vi "Request - Parse Header.vi"() -> (3 "Unit Test Framework Results":T1)   [LabVIEW 2023, in "Request.lvclass"]
doc: "Use this template to create a user-defined test VI. Define your test requirements and wire the results to the <b>Result (Test)</b> control. Do not modify the <b>Unit Test Framework Results</b> indicator."
uses:
  Request.lvclass
  <vilib>/utf/common/utf_test_comparison_operators.ctl
  <vilib>/utf/NI_UnitTestFramework.lvlib
  <vilib>/utf/common/utf_test_result.ctl
  <vilib>/utf/common/utf_test_result_failure.ctl
  <vilib>/utf/common/utf_test_result_troll.ctl
  <vilib>/utf/common/utf_vi_tag.ctl
  Request.ctl
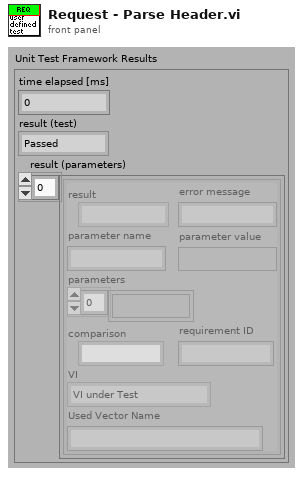
[diagram p1: front panel]
types:
  T1 = typedef "NI_UnitTestFramework.lvlib/utf_test_result_troll.ctl" = cluster{"time elapsed [ms]":u32, "result (test)":T2, "result (parameters)":T3[]}
  T2 = typedef "NI_UnitTestFramework.lvlib/utf_test_result.ctl" = enum16{"Passed", "Failed", "Error", "Skipped", "Not Processed"}
  T3 = typedef "NI_UnitTestFramework.lvlib/utf_test_result_failure.ctl" = cluster{"result":T2, "error message":string, "parameter name":string, "parameter value":variant, "parameters":variant[], "comparison":T4, "requirement ID":string, "VI":T5, "Used Vector Name":string}
  T4 = typedef "NI_UnitTestFramework.lvlib/utf_test_comparison_operators.ctl" = enum16{"=", "!=", ">", ">=", "<", "<=", "range", "symmetric tolerance", "asymmetric tolerance", "string contains", "string not contain", "array size", "string length", "array range", "by element", "array range (limit array)", "user-defined", "array contains", "array not contain", "vector length", "= (elm)", "!= (elm)", "= (case insensitive)", "!= (case insensitive)"}
  T5 = typedef "NI_UnitTestFramework.lvlib/utf_vi_tag.ctl" = enum16{"Setup VI", "VI under Test", "Teardown VI"}
  T6 = typedef "Request.ctl" = cluster{"Method":string, "URI":string, "Protocol":string, "Raw Path":string, "Query":string, "Fragment":string, "Raw Body":string, "Headers":variant, "Parameters":variant, "Body":variant, "Raw Header":string, "Path":string[]}
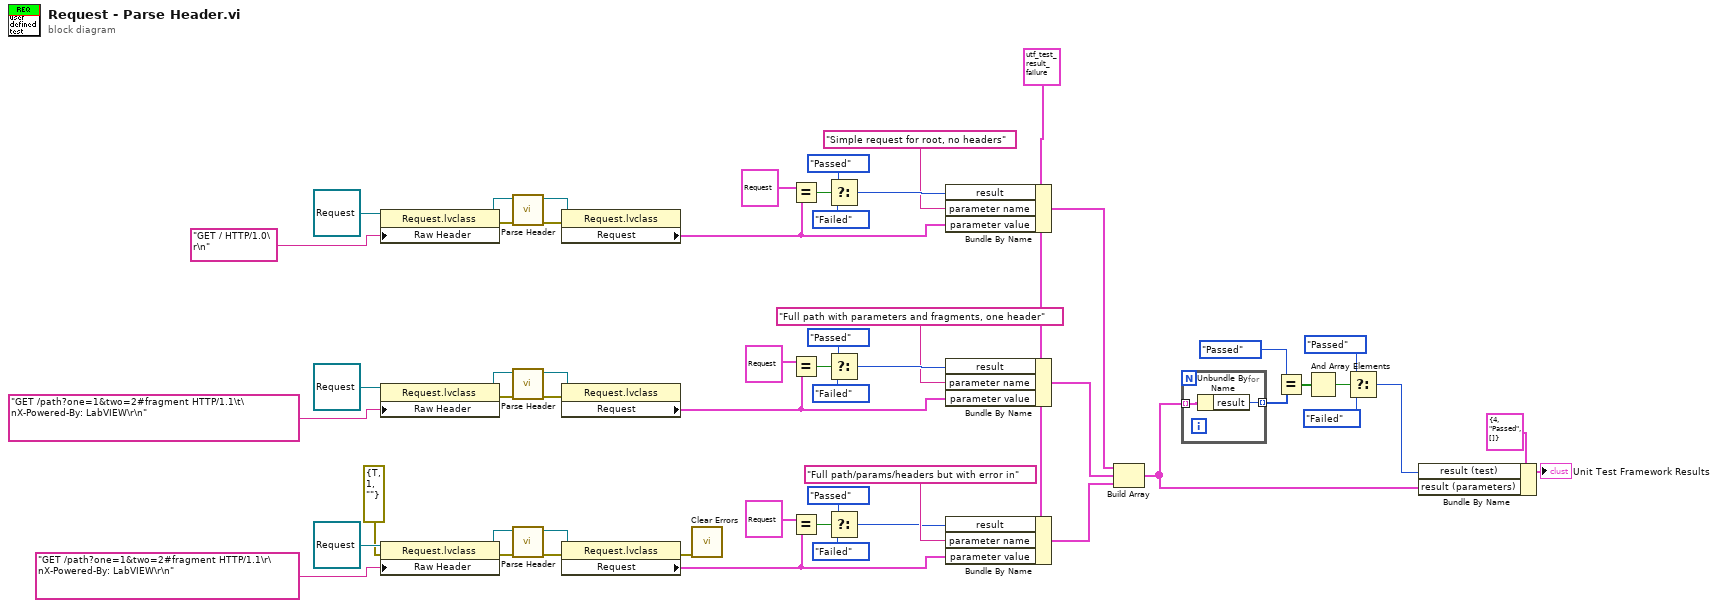
[diagram p0: block diagram]
diagram:
  w9 = T3 {"result"=enum."Not Processed", "error message"="", "parameter name"="", "parameter value"=variant, "parameters"=[], "comparison"=enum."=", "requirement ID"="", "VI"=enum."VI under Test", "Used Vector Name"=""} ("Unit Test Framework - result (parameters)")
  n1 = property class="Request.lvclass"(reference=refnum<class "Request.lvclass"> refnum ("Request.lvclass"), "Raw Header"="GET / HTTP/1.0\r\n") -> (reference out=w52:refnum<class "Request.lvclass">, error out=w51:errorcluster)  [unwired: 1 in]
  n2 = property class="Request.lvclass"(reference=refnum<class "Request.lvclass"> refnum ("Request.lvclass"), "Raw Header"="GET /path?one=1&two=2#fragment HTTP/1.1\t\nX-Powered-By: LabVIEW\r\n") -> (reference out=w30:refnum<class "Request.lvclass">, error out=w31:errorcluster)  [unwired: 1 in]
  n3 = property class="Request.lvclass"(reference=refnum<class "Request.lvclass"> refnum ("Request.lvclass"), error in=errorcluster {"status"=TRUE, "code"=1, "source"=""} ("error in (no error)"), "Raw Header"="GET /path?one=1&two=2#fragment HTTP/1.1\r\nX-Powered-By: LabVIEW\r\n") -> (reference out=w15:refnum<class "Request.lvclass">, error out=w14:errorcluster)
  n4 = call "Parse Header.vi"("error in (no error)"=w51, "Request in"=w52) -> ("error out"=w50:errorcluster, "Request out"=w49:refnum<class "Request.lvclass">)  [unwired: 8 in]
  n5 = call "Parse Header.vi"("error in (no error)"=w31, "Request in"=w30) -> ("error out"=w32:errorcluster, "Request out"=w33:refnum<class "Request.lvclass">)  [unwired: 8 in]
  n6 = call "Parse Header.vi"("error in (no error)"=w14, "Request in"=w15) -> ("error out"=w13:errorcluster, "Request out"=w12:refnum<class "Request.lvclass">)  [unwired: 8 in]
  n7 = property class="Request.lvclass"(reference=w49, error in=w50) -> ("Request"=w4:T6)  [unwired: 2 out]
  n8 = property class="Request.lvclass"(reference=w33, error in=w32) -> ("Request"=w6:T6)  [unwired: 2 out]
  n9 = property class="Request.lvclass"(reference=w12, error in=w13) -> (error out=w7:errorcluster, "Request"=w5:T6)  [unwired: 1 out]
  n10 = call <vilib>:"Clear Errors.vi"("error in (no error)"=w7) -> ()  [unwired: 5 in, 2 out]
  n11 = Equal?(x=T6 {"Method"="GET", "URI"="/", "Protocol"="HTTP/1.0", "Raw Path"="/", "Query"="", "Fragment"="", "Raw Body"="", "Headers"=variant, "Parameters"=variant, "Body"=variant, "Raw Header"="GET / HTTP/1.0\r\n", "Path"=[""]} ("Request"), y=w4) -> (x = y?=w35:bool)
  n12 = Equal?(x=T6 {"Method"="GET", "URI"="/path?one=1&two=2#fragment", "Protocol"="HTTP/1.1\t\nX-Powered-By:", "Raw Path"="/path?one=1&two=2", "Query"="one=1&two=2", "Fragment"="fragment", "Raw Body"="", "Headers"=variant, "Parameters"=variant("one"=variant(string "1"), "two"=variant(string "2")), "Body"=variant, "Raw Header"="GET /path?one=1&two=2#fragment HTTP/1.1\t\nX-Powered-By: LabVIEW\r\n", "Path"=["path"]} ("Request 2"), y=w6) -> (x = y?=w28:bool)
  n13 = Equal?(x=T6 {"Method"="", "URI"="", "Protocol"="", "Raw Path"="", "Query"="", "Fragment"="", "Raw Body"="", "Headers"=variant, "Parameters"=variant, "Body"=variant, "Raw Header"="", "Path"=[]} ("Request 3"), y=w5) -> (x = y?=w17:bool)
  n14 = Select(t=utf_test_result."Passed" ("result"), s=w35, f=utf_test_result."Failed" ("result")) -> (s? t:f=w47:T2)
  n15 = Select(t=utf_test_result."Passed" ("result"), s=w28, f=utf_test_result."Failed" ("result")) -> (s? t:f=w25:T2)
  n16 = Select(t=utf_test_result."Passed" ("result"), s=w17, f=utf_test_result."Failed" ("result")) -> (s? t:f=w20:T2)
  n17 = Bundle By Name(cluster=w9, "result"=w47, "parameter name"="Simple request for root, no headers", "parameter value"=w4) -> (w48:T3)
  n18 = Bundle By Name(cluster=w9, "result"=w25, "parameter name"="Full path with parameters and fragments, one header", "parameter value"=w6) -> (w24:T3)
  n19 = Bundle By Name(cluster=w9, "result"=w20, "parameter name"="Full path/params/headers but with error in", "parameter value"=w5) -> (w10:T3)
  n20 = Build Array(w48, w24, w10) -> (w44:T3[])
  n21 = for {
    tunnel: w44 -> [w57] mode=indexing
    tunnel: [w56] -> w43 mode=indexing
    n22 = Unbundle By Name(w57) -> ("result"=w56:T2)
  }
  n23 = Equal?(x=utf_test_result."Passed" ("result"), y=w43) -> (x = y?=w41:bool[])
  n24 = And Array Elements(Boolean array=w41) -> (logical AND=w40:bool)
  n25 = Select(t=utf_test_result."Passed" ("result"), s=w40, f=utf_test_result."Failed" ("result")) -> (s? t:f=w37:T2)
  n26 = Bundle By Name(cluster=T1 {"time elapsed [ms]"=4, "result (test)"=enum."Passed", "result (parameters)"=[]} ("Unit Test Framework - Result"), "result (test)"=w37, "result (parameters)"=w44) -> (→"Unit Test Framework Results":T1)
